vi "Capacitance_IS_CalculateZRef.vi"(7 "Data Id":string, 9 "ZCal":dbl, 10 "FGEN Parameters":T2 {"Trigger Mode" items=["Single", "Continuous", "Stepped", "Burst"]}, 11 "Semiconductor Module Context":T1) -> (0 "error out":errorcluster, 2 "Frequencies":dbl[](array[numeric]), 3 "ZRef":cdb[](array[numeric]))   [LabVIEW 2023, in "Capacitance.lvlib"]
doc: "Calculates ZRef= ZCal*V2/(V1-V2) using the V1 and V2 FFT results measured"
uses:
  Capacitance.lvlib
  ResourceHandling/TypeDefs/RH_FGEN_Parameters.ctl
  <instrlib>/niFgen/niFgen.llb/niFgen Trigger Mode.ctl
  <vilib>/NI_TestStand_SemiconductorModule/NI_TestStand_Semiconductor_Module.lvlibp/PinMap/General/SemiconductorModuleContext.ctl
  <vilib>/Analysis/1siggen.llb/Ramp Pattern by Delta.vi
  Resonance/Resonance.lvlib
  <vilib>/Analysis/NI_AALBase.lvlib
  <vilib>/NI_TestStand_SemiconductorModule/NI_TestStand_Semiconductor_Module.lvlibp
  ResourceHandling/ResourceHandling.lvlib
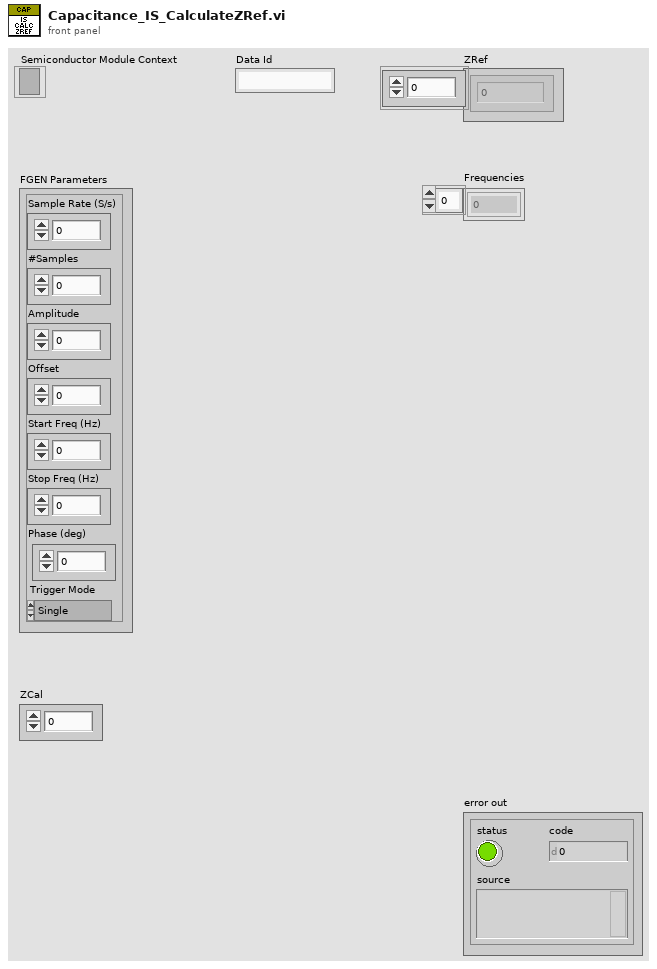
[diagram p1: front panel]
types:
  T1 = typedef "NI_TestStand_Semiconductor_Module.lvlibp/SemiconductorModuleContext.ctl" = refnum<k7>
  T2 = typedef "ResourceHandling.lvlib/RH_FGEN_Parameters.ctl" = cluster{"Sample Rate (S/s)":dbl, "#Samples":i32, "Amplitude":dbl, "Offset":dbl, "Start Freq (Hz)":dbl, "Stop Freq (Hz)":dbl, "Phase (deg)":dbl, "Trigger Mode":T3}
  T3 = typedef "niFgen Trigger Mode.ctl" = i32
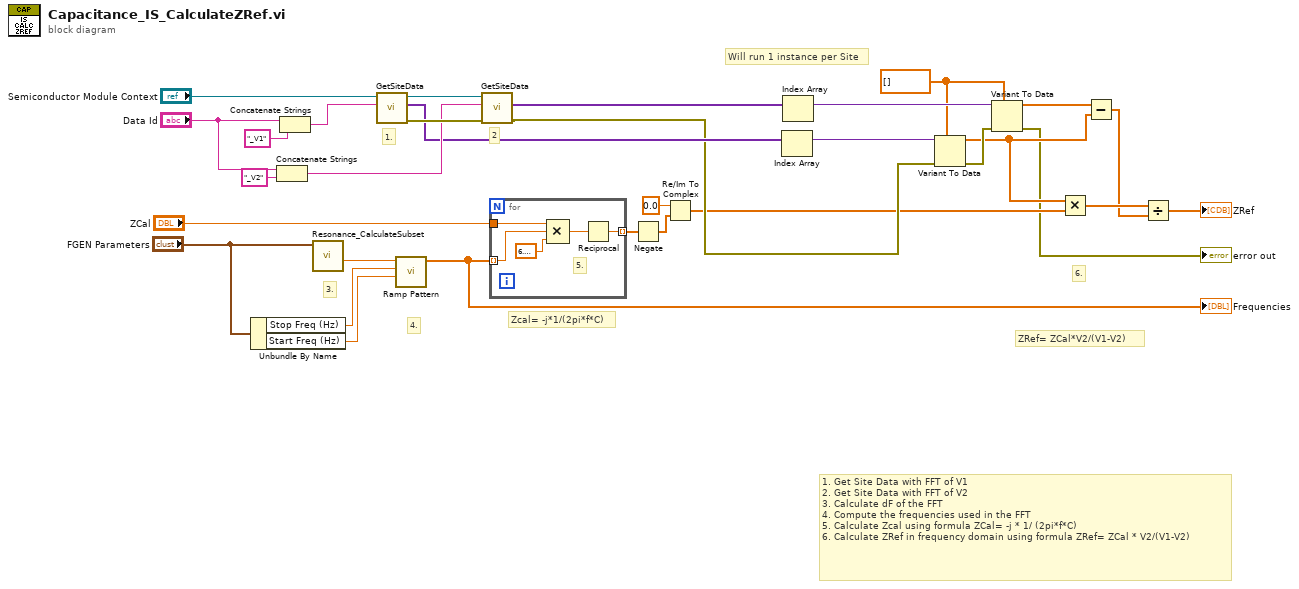
[diagram p0: block diagram]
diagram:
  w7 = cdb[] []
  # "6."
  # "Will run 1 instance per Site"
  # "1. Get Site Data with FFT of V1\n2. Get Site Data with FFT of V2\n3. Calculate dF of the FFT\n4. Compute the frequencies used in the FFT \n5. Calculate Zcal using formula ZCal= -j * 1/ (2pi*f*C)\n6. Calculate ZRef in frequency domain using formula ZRef= ZCal * V2/(V1-V2)"
  # "2"
  # "1."
  # "4."
  # "3."
  # "ZRef= ZCal*V2/(V1-V2)"
  # "Zcal= -j*1/(2pi*f*C)"
  n1 = Unbundle By Name("FGEN Parameters") -> ("Stop Freq (Hz)"=w29:dbl, "Start Freq (Hz)"=w28:dbl)
  n2 = Concatenate Strings("Data Id", "_V2" ("string")) -> (w20:string)
  n3 = Concatenate Strings("Data Id", "_V1" ("string")) -> (w25:string)
  n4 = call "Resonance_CalculateSubset.vi"("FGEN Parameters"="FGEN Parameters") -> ("dF"=w31:dbl)  [unwired: 6 in, 4 out]
  n5 = call <vilib>:"GetSiteData.vi"("Data Id"=w25, "Semiconductor Module Context"="Semiconductor Module Context") -> ("error out"=w23:errorcluster, "Site Data"=w18:variant[], "Semiconductor Module Context Out"=w24:T1)  [unwired: 7 in]
  n6 = call-poly <vilib>:"Ramp Pattern.vi"("start"=w28, "end"=w29, "delta"=w31) -> ("Ramp Pattern"=w12:dbl[])  [unwired: 6 in, 2 out]
  "Frequencies" <- w12
  n7 = call <vilib>:"GetSiteData.vi"("error in (no error)"=w23, "Data Id"=w20, "Semiconductor Module Context"=w24) -> ("error out"=w17:errorcluster, "Site Data"=w19:variant[])  [unwired: 6 in, 1 out]
  n8 = for {
    tunnel: w12 -> [w35] mode=indexing
    tunnel: "ZCal" -> [w36]
    tunnel: [w32] -> w15 mode=indexing
    # "5."
    n9 = Compound Arithmetic op=MULTIPLY(w36, w35, 6.283185307179586) -> (w33:dbl)
    n10 = Reciprocal(x=w33) -> (1/x=w32:dbl)
  }
  n11 = Negate(x=w15) -> (-x=w14:dbl[])
  n12 = Re/Im To Complex(1:w14, 2:0.0 ("x")) -> (0:w13:cdb[])
  n13 = Index Array(array=w18) -> (element=w9:variant)  [unwired: 1 in]
  n14 = Index Array(array=w19) -> (element=w10:variant)  [unwired: 1 in]
  n15 = Variant To Data(error in=w17, type=w7, Variant=w9) -> (data=w5:cdb[], error out=w8:errorcluster)
  n16 = Variant To Data(error in=w8, type=w7, Variant=w10) -> (data=w6:cdb[], error out=→"error out":errorcluster)
  n17 = Multiply(x=w5, y=w13) -> (x*y=w4:cdb[])
  n18 = Subtract(x=w6, y=w5) -> (x-y=w3:cdb[])
  n19 = Divide(x=w4, y=w3) -> (x/y=→"ZRef":cdb[])
